vi "Autofocus.vi"() -> ()   [LabVIEW 2015]
uses:
  <vilib>/vision/Image Controls.llb/IMAQ Image.ctl
  <vilib>/Platform/TimedLoop/XDataNode/timing_clust.ctl
  <vilib>/Platform/TimedLoop/XDataNode/nitl_modes.ctl
  <vilib>/Platform/TimedLoop/XDataNode/wakeup.ctl
  <vilib>/platform/TimedLoop/XDataNode/XDataNode.xnode
  <vilib>/vision/NI_Vision_Development_Module.lvlib
  <vilib>/Platform/TimedLoop/XDataNode/XDNodeRunTimeDep.lvlib
panel:
  in  "P":dbl
  out "ImageDistances":dbl[](graph)
  out "Waveform Chart":i32(graph)
  in  "Pause?":bool
  out "decision":i32
  out "Y Resolution 2":i32
  out "X Resolution 2":i32
  out "average image buffer":T1[](array[typedef])
  out "Z autofocus distance":dbl=nan
  in  "Step size (um)":dbl
  in  "Capture BG":bool
  out "Distance":dbl=nan
  in  "Scan":bool
  out "Paused":bool
  in  "Threshold":dbl
  in  "Measure And Track":bool
  in  "Control Z":string="Off"
  out "Moving":bool
  out "error out":errorcluster
  out "Actual position":dbl[](array[numeric])=[49.9991798, 49.9997406, 53.0021973] format="%.6f"
  in  "Pi System No":i32=1
  in  "Position":cluster{"X":dbl, "Y":dbl, "Z":dbl}={"X"=50.0, "Y"=50.0, "Z"=50.0} {"Z" min=0.0 max=1000.0 step=0.001 format="%5.3g"; "Y" min=0.0 max=100.0 step=0.001 format="%06.3g"; "X" min=0.0 max=100.0 step=0.001 format="%05.3g"}
  in  "stop 2":bool
  out "Running":bool=TRUE caption="Configuration_Setup.vi is running"
  out "Conn. Axis":string[](array[string])=["1", "2", "3"]
  out "Identification":string="Physik Instrumente, E-725, 112059106, 12.01.04.04"
  in  "Z_ROI":i32[](array[numeric])=[0, 2, 10, 10]
  out "Micrograph":T1(plugin-control)
  in  "stop":bool
  # "Piezo Control"
  # "Z axis autofocus"
  # "Debug"
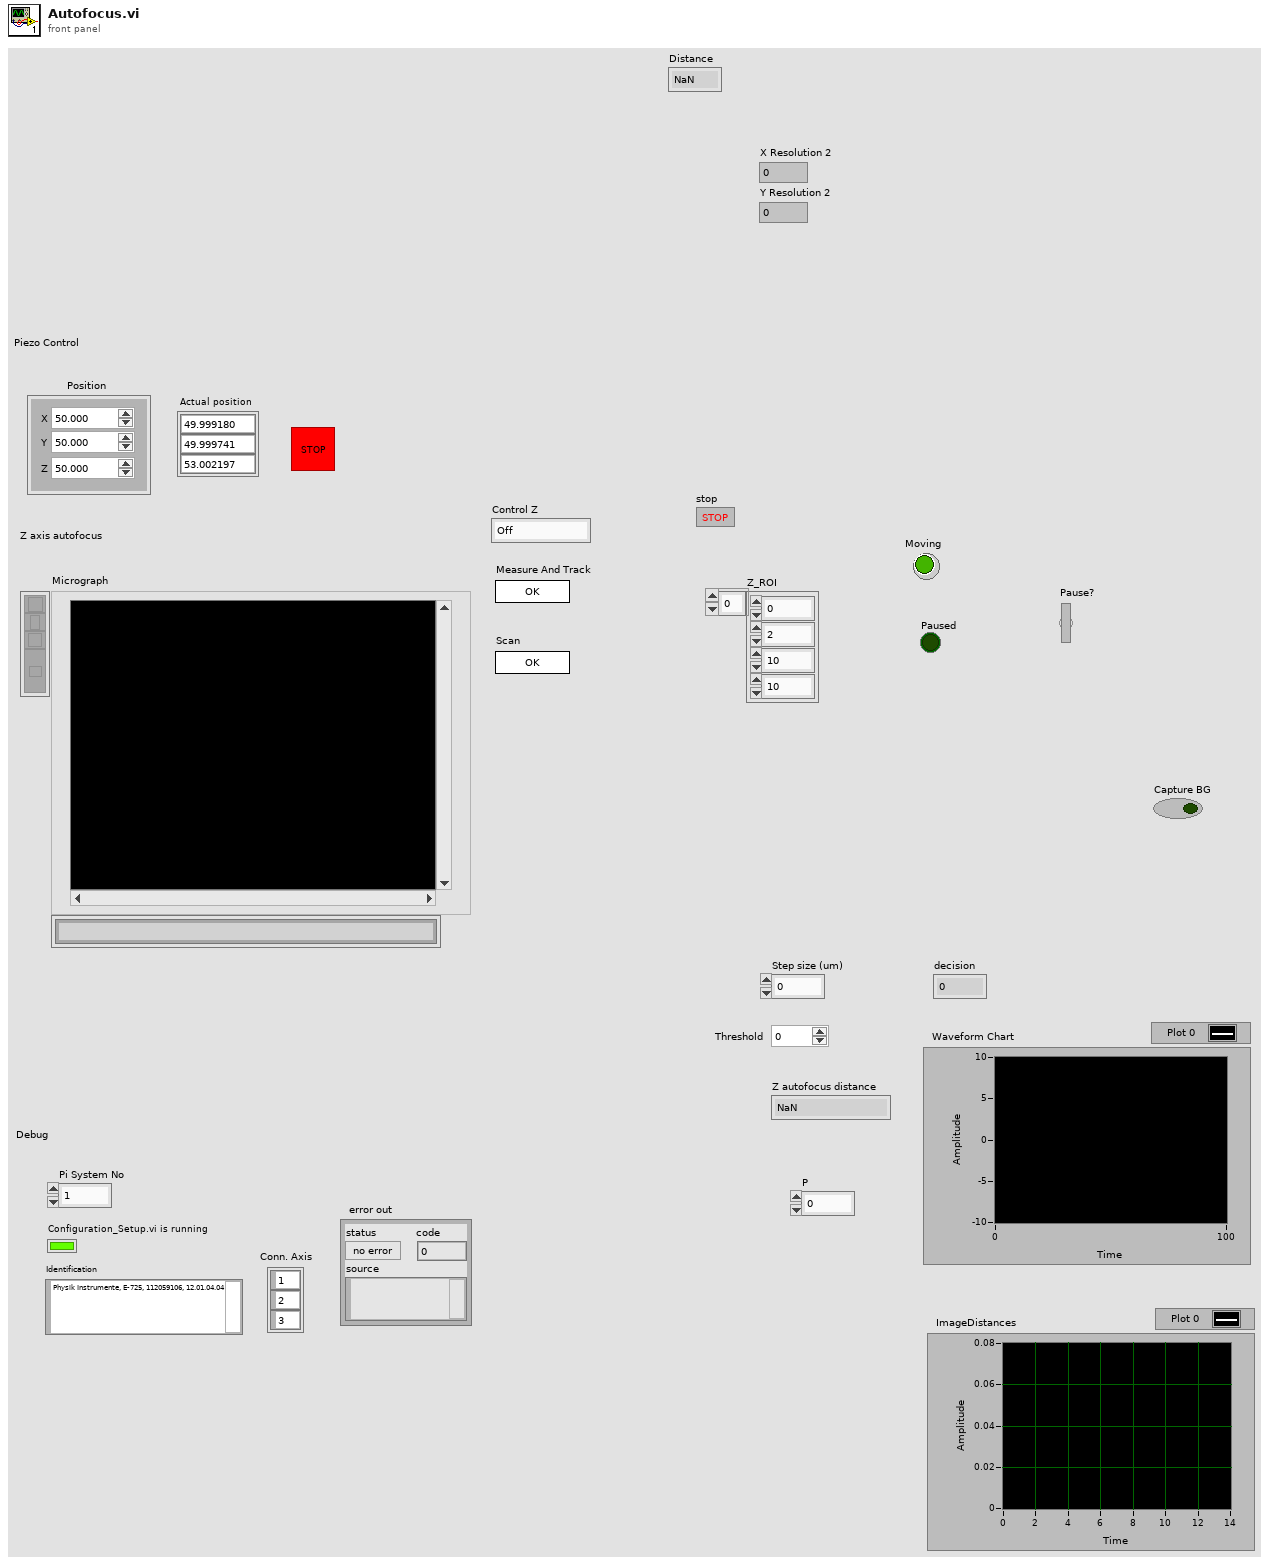
[diagram p1: front panel]
types:
  T1 = typedef "IMAQ Image.ctl" = refnum<image>
  T2 = typedef "XDNodeRunTimeDep.lvlib/timing_clust.ctl" = cluster{"Expected End [f-1]":u64, "Actual End [f-1]":u64, "Finished Late? [f-1]":bool, "Expected End [i-1]":u64, "Actual End [i-1]":u64, "Finished Late? [i-1]":bool, "Expected Start [i]":u64, "Actual Start [i]":u64, "Expected Start [f]":u64, "Actual Start [f]":u64, "Source Name":string, "Structure Name":string, "Period":i64, "Deadline":i64, "Offset":i64, "Start":i64, "Priority":i32, "Timeout":i32, "Mode":T3, "Wakeup Reason":T4, "Error":errorcluster, "Source Type":string, "Secondary Source Type":string, "Global End Time":u64, "Global Start Time":u64, "Frame Duration":u64, "Iteration Duration":u64, "Assigned CPU":i32, "I/O Scan Engine Mode":u32}
  T3 = typedef "XDNodeRunTimeDep.lvlib/nitl_modes.ctl" = enum32{"No Change", "Process missed periods, maintain original phase", "Discard missed periods, maintain original phase", "Process missed periods, ignore original phase", "Discard missed periods, ignore original phase"}
  T4 = typedef "XDNodeRunTimeDep.lvlib/wakeup.ctl" = enum32{"Normal", "Aborted", "Asynchronous wakeup", "Timing source error", "Timed loop error", "Timeout"}
  T5 = cluster{"Global Rectangle":i32[], "Contours":cluster{"Contour Type":u32, "ROI Type":u32, "Points":i32[]}[]}
  T6 = typedef "ROI Descriptor" = cluster{"Global Rectangle":i32[], "Contours":cluster{"ID":enum32{"External", "Internal"}, "Type":u32, "Coordinates":i32[]}[]}
  T7 = typedef "IMAQ Point" = cluster{"X":sgl, "Y":sgl}
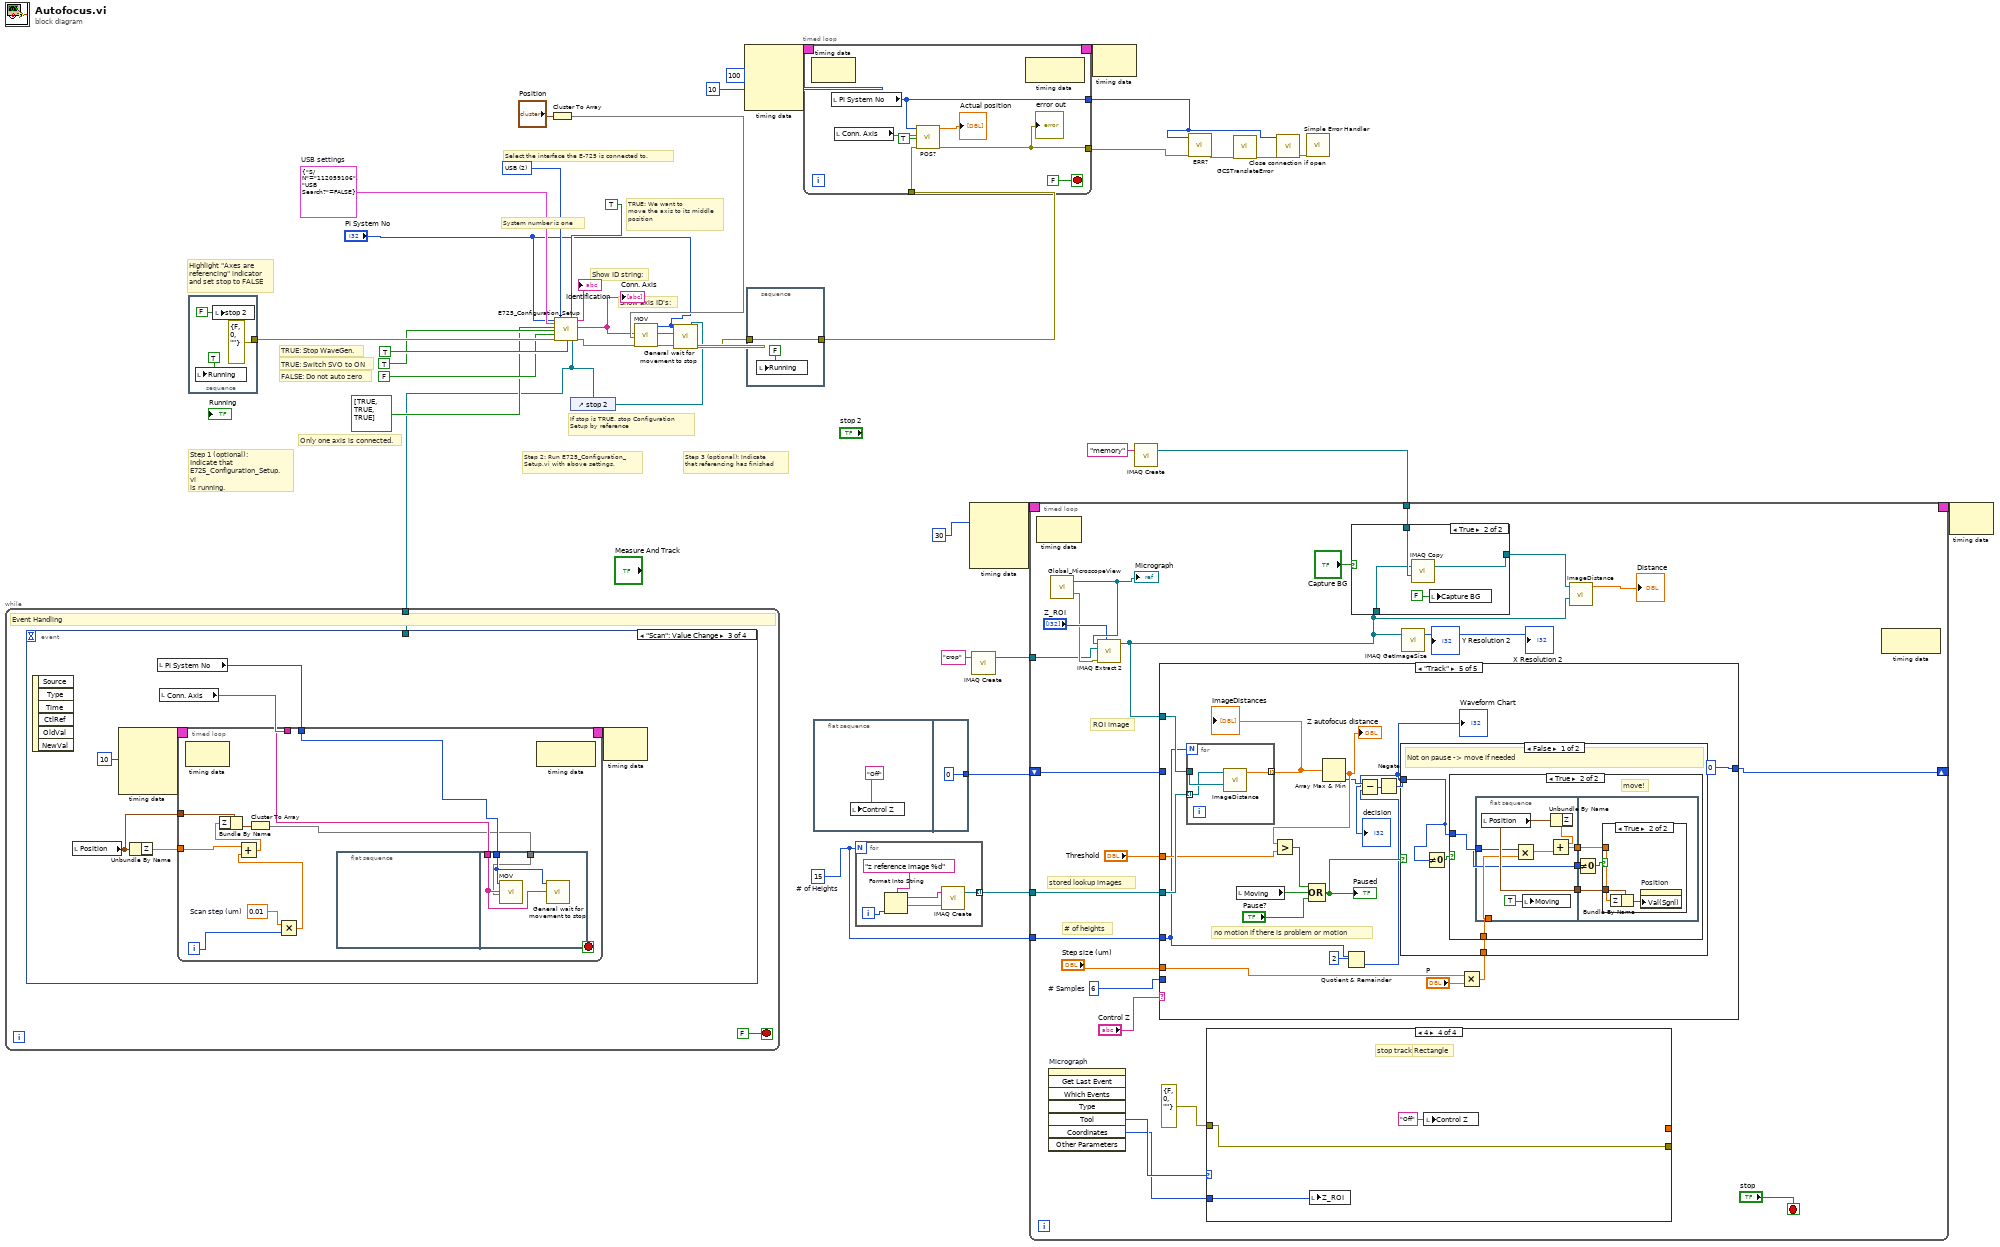
[diagram p0: block diagram]
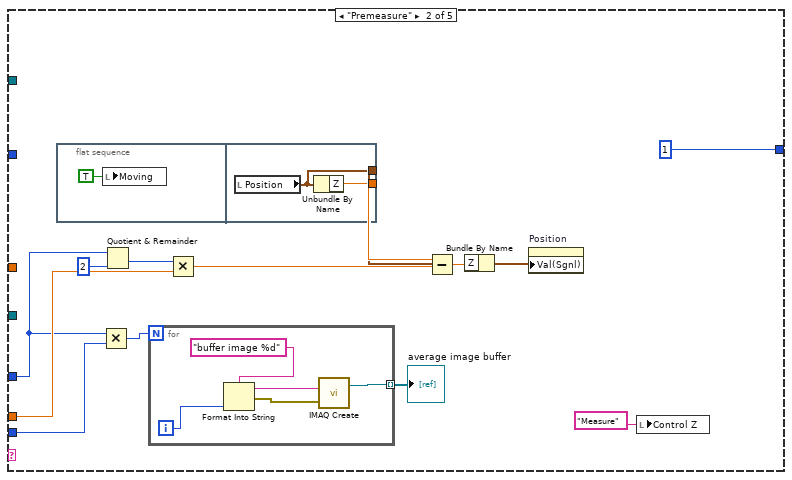
[diagram p4: hidden frame]
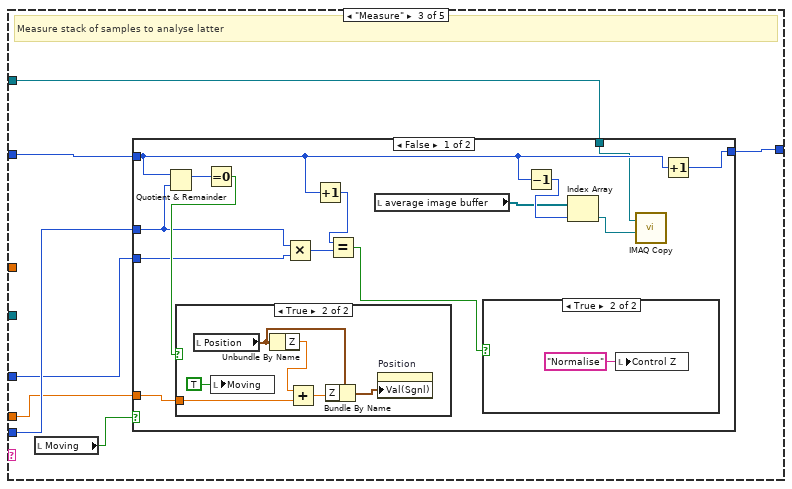
[diagram p5: hidden frame]
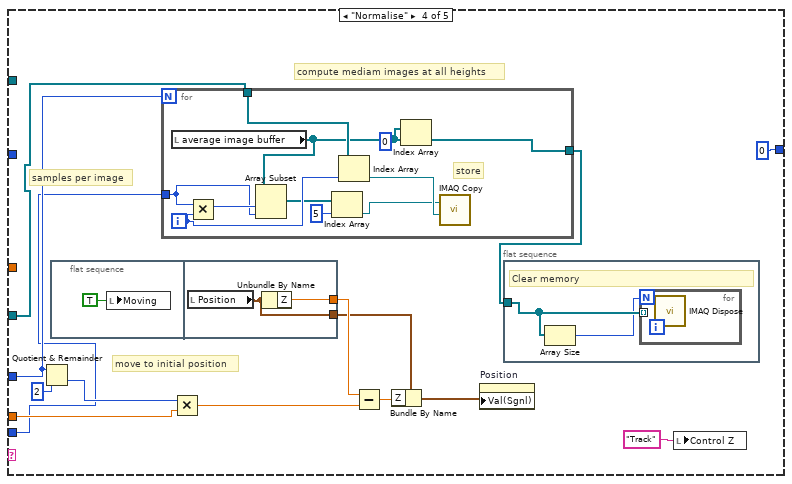
[diagram p9: hidden frame]
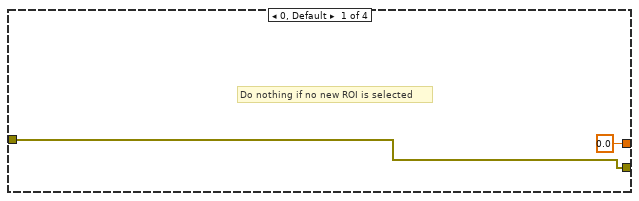
[diagram p13: hidden frame]
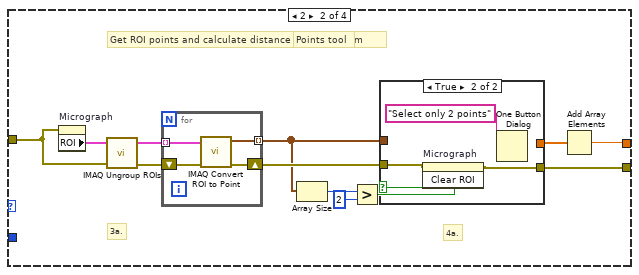
[diagram p14: hidden frame]
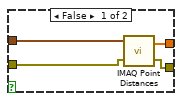
[diagram p15: hidden frame]
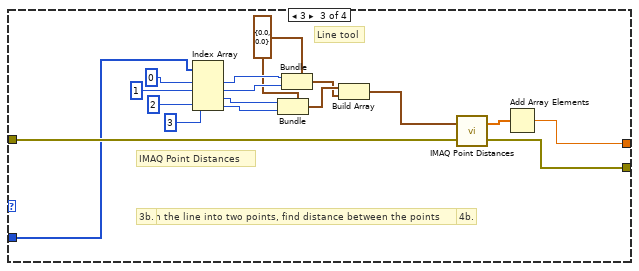
[diagram p16: hidden frame]
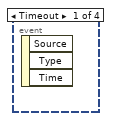
[diagram p17: hidden frame]
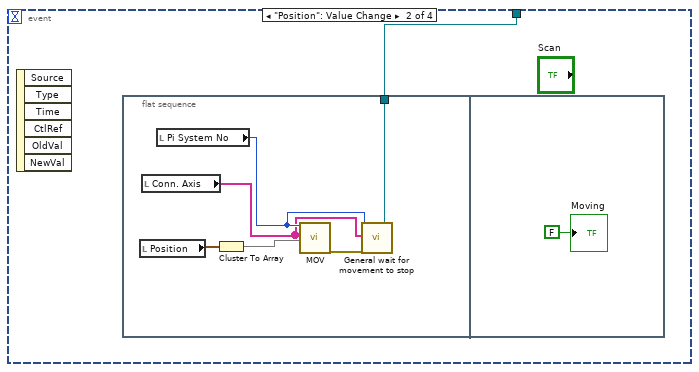
[diagram p18: hidden frame]
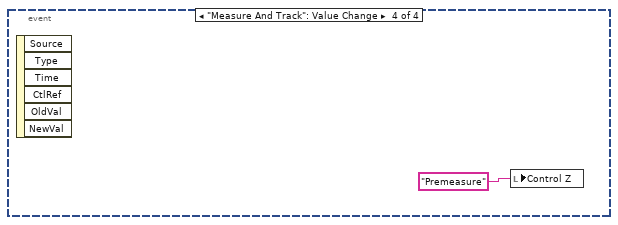
[diagram p19: hidden frame]
diagram:
  w1 = 15  # # of Heights
  w30 = cluster{"S/N":string, "USB Search?":bool} {"S/N"="112059106", "USB Search?"=FALSE}  # USB settings
  w21 = u16 2 items=["RS232", "TCP/IP", "USB"] ("Interface")
  # "Only one axis is connected."
  # "TRUE: We want to\nmove the axis to its middle\nposition"
  # "FALSE: Do not auto zero"
  # "TRUE: Switch SVO to ON"
  # "If stop is TRUE, stop Configuration\nSetup by reference"
  # "Select the interface the E-725 is connected to."
  # "Step 3 (optional): Indicate\nthat referencing has finished"
  # "Step 2: Run E725_Configuration_\nSetup.vi with above settings."
  # "Step 1 (optional): \nIndicate that\nE725_Configuration_Setup.vi\nis running."
  # "Highlight \"Axes are\nreferencing\" indicator\nand set stop to FALSE"
  # "Show axis ID's:"
  # "Show ID string:"
  # "TRUE: Stop WaveGen."
  # "System number is one"
  n1 = stacked-sequence {
    tunnel: [errorcluster {"status"=FALSE, "code"=0, "source"=""} ("error in")] -> w36
    frame #0 {
      n2 = local write "Running"(TRUE ("Running")) -> ()
      n3 = local write "stop 2"(FALSE ("stop")) -> ()
    }
  }
  n4 = Cluster To Array(cluster="Position") -> (array=w24:dbl[])
  n5 = control-ref of="stop 2"() -> (w14:refnum<vi>)
  n6 = while {
    tunnel: w14 -> [w42]
    stop <- FALSE stop-if-true
    # "Event Handling"
    n7 = event shown="[2] \"Scan\": Value Change" {
      selector: _ -> [_ _ _ _]
      dyn-events: _ -> [_ _ _ _]
      timeout: _ -> [_ _ _ _]
      tunnel: w42 -> [_ w43 _ _]
      event Timeout {
        n8 = event-data() -> ()  [unwired: 1 in, 3 out]
      }
      event "Position": Value Change {
        n9 = event-data() -> ()  [unwired: 1 in, 6 out]
        n10 = flat-sequence {
          tunnel: w43 -> [w44]
          frame #0 {
            n11 = local read "Position"() -> (w49:cluster{"X":dbl, "Y":dbl, "Z":dbl})
            n12 = local read "Conn. Axis"() -> (w45:string[])
            n13 = local read "Pi System No"() -> (w46:i32)
            n14 = Cluster To Array(cluster=w49) -> (array=w48:dbl[])
            n15 = call "MOV.vi"("System no."=w46, "Axes to move"=w45, "Position values"=w48) -> ("error out"=w47:errorcluster)  [unwired: 16 in]
            n16 = call "General wait for movement to stop.vi"("System no."=w46, "Axes to wait for"=w45, "error in"=w47, "Stop refnum"=w44) -> ()  [unwired: 14 in, 2 out]
          }
          frame #1 {
            "Moving" <- FALSE
          }
        }
      }
      event "Scan": Value Change {
        n17 = event-data() -> ()  [unwired: 1 in, 6 out]
        n18 = local read "Position"() -> (w53:cluster{"X":dbl, "Y":dbl, "Z":dbl})
        n19 = node-c288(i64 10 ("Period")) -> (w56:T2)  [unwired: 3 in]
        n20 = Unbundle By Name(w53) -> ("Z"=w57:dbl)
        n21 = local read "Pi System No"() -> (w51:i32)
        n22 = local read "Conn. Axis"() -> (w52:string[])
        n23 = timed-loop {
          tunnel: w57 -> [w65]
          timing: w56 -> [_]
          timing-out: [_] -> w55
          tunnel: w53 -> [w63]
          tunnel: w52 -> [w59]
          tunnel: w51 -> [w60]
          i -> [w66]
          stop <- _ stop-if-true
          w67 = 0.01  # Scan step (um)
          n24 = node-c288() -> ()  [unwired: 1 in, 1 out]
          n25 = Multiply(x=w67, y=w66) -> (x*y=w64:dbl)
          n26 = Add(x=w65, y=w64) -> (x+y=w61:dbl)
          n27 = Bundle By Name(cluster=w63, "Z"=w61) -> (w62:cluster{"X":dbl, "Y":dbl, "Z":dbl})
          n28 = Cluster To Array(cluster=w62) -> (array=w58:dbl[])
          n29 = flat-sequence {
            tunnel: w60 -> [w70]
            tunnel: w59 -> [w69]
            tunnel: w58 -> [w68]
            frame #0 {
            }
            frame #1 {
              n30 = call "MOV.vi"("System no."=w70, "Axes to move"=w69, "Position values"=w68) -> ()  [unwired: 16 in, 1 out]
              n31 = call "General wait for movement to stop.vi"("System no."=w70, "Axes to wait for"=w69) -> ()  [unwired: 16 in, 2 out]
            }
          }
          n32 = node-c288() -> ()  [unwired: 1 in, 1 out]
        }
        n33 = node-c288(w55) -> ()  [unwired: 1 out]
      }
      event "Measure And Track": Value Change {
        n34 = event-data() -> ()  [unwired: 1 in, 6 out]
        n35 = local write "Control Z"("Premeasure" ("Control Z")) -> ()
      }
    }
  }
  n36 = call "E725_Configuration_Setup.vi"("System no."="Pi System No", "USB settings"=w30, "Are stages connected?"=bool[] [TRUE, TRUE, TRUE], "Change servo status to ON?"=TRUE ("Use dialog to define\nconnected stages?"), "Perform autozero?"=FALSE ("Use dialog to define\nconnected stages?"), "error in"=w36, "Interface"=w21, "Stop wave generator\noutput (if any)"=TRUE ("All axes?"), "Move to middle?"=TRUE, "Stop refnum"=w14) -> ("Identification"=→"Identification":string, "All conn. axes"=w20:string[], "error out"=w26:errorcluster)  [unwired: 5 in, 2 out]
  "Conn. Axis" <- w20
  n37 = call "MOV.vi"("System no."="Pi System No", "Axes to move"=w20, "Position values"=w24, "error in"=w26) -> ("error out"=w23:errorcluster)  [unwired: 15 in]
  n38 = call "General wait for movement to stop.vi"("System no."="Pi System No", "Axes to wait for"=w20, "error in"=w23, "Stop refnum"=w14) -> ("error out"=w22:errorcluster)  [unwired: 14 in, 1 out]
  n39 = node-c288(i64 100 ("Period"), 10 ("Priority")) -> (w19:T2)  [unwired: 2 in]
  n40 = stacked-sequence {
    tunnel: w22 -> [w79]
    tunnel: [w79] -> w15
    frame #0 {
      n41 = local write "Running"(FALSE ("Running")) -> ()
    }
  }
  n42 = timed-loop {
    timing: w19 -> [_]
    timing-out: [_] -> w18
    tunnel: w15 -> [w85]
    tunnel: [w81] -> w12
    tunnel: [w80] -> w13
    stop <- FALSE stop-if-true
    n43 = node-c288() -> ()  [unwired: 1 in, 1 out]
    n44 = local read "Pi System No"() -> (w80:i32)
    n45 = local read "Conn. Axis"() -> (w84:string[])
    n46 = call "POS?.vi"("System no."=w80, "Axes to query"=w84, "All axes?"=TRUE, "error in"=w85) -> ("Position"=→"Actual position":dbl[], "error out"=w81:errorcluster)  [unwired: 14 in]
    "error out" <- w81
    n47 = node-c288() -> ()  [unwired: 1 in, 1 out]
  }
  n48 = flat-sequence {
    tunnel: [0] -> w7
    frame #0 {
      n49 = local write "Control Z"("Off" ("Control Z")) -> ()
    }
    frame #1 {
    }
  }
  n50 = for {
    N: w1 -> [_]
    tunnel: [w95] -> w3 mode=indexing
    i -> [w93]
    n51 = Format Into String(format string="z reference image %d", w93) -> (resulting string=w91:string, error out=w92:errorcluster)  [unwired: 2 in]
    n52 = call "IMAQ Create"("Image Name"=w91, "error in (no error)"=w92) -> ("New Image"=w95:T1)  [unwired: 3 in, 1 out]
  }
  n53 = node-c288(i64 30 ("Period")) -> (w10:T2)  [unwired: 3 in]
  n54 = call "IMAQ Create"("Image Name"="crop") -> ("New Image"=w2:T1)  [unwired: 4 in, 1 out]
  n55 = node-c288(w18) -> ()  [unwired: 1 out]
  n56 = call "IMAQ Create"("Image Name"="memory") -> ("New Image"=w4:T1)  [unwired: 4 in, 1 out]
  n57 = timed-loop {
    timing: w10 -> [_]
    timing-out: [_] -> w9
    shift-right: [w114] -> _
    shift-left: w7 -> [w113]
    tunnel: w4 -> [w108]
    tunnel: w3 -> [w103]
    tunnel: w2 -> [w101]
    tunnel: w1 -> [w99]
    stop <- "stop" stop-if-true
    w112 = 6  # # Samples
    # "stored lookup images"
    # "# of heights"
    # "ROI image"
    n58 = node-c288() -> ()  [unwired: 1 in, 1 out]
    n59 = invoke on="Micrograph" class="ImageControl" method="Get Last Event"() -> ("Tool"=w117:i32, "Coordinates"=w116:i32[])  [unwired: 8 in, 6 out]
    n60 = call "Global_MicroscopeView.vi"() -> ("error out"=w102:errorcluster, "MicroscopeView"=w109:T1)  [unwired: 4 in]
    "Micrograph" <- w109
    n61 = call "IMAQ Extract 2"("Optional Rectangle"="Z_ROI", "error in (no error)"=w102, "Image Dst"=w101, "Image Src"=w109) -> ("Image Dst Out"=w98:T1)  [unwired: 6 in, 1 out]
    n62 = case shown="\"Track\"" "Control Z" {
      tunnel: [w124 1 w152 0 0] -> w114
      tunnel: w113 -> [w124 _ w153 _ _]
      tunnel: w112 -> [_ w126 w151 w178 _]
      tunnel: "Step size (um)" -> [_ w135 w150 w185 w210]
      tunnel: "Threshold" -> [_ _ _ _ w221]
      tunnel: w103 -> [_ _ _ w177 w222]
      tunnel: w98 -> [_ _ w147 _ w223]
      tunnel: w99 -> [_ w125 w148 w179 w213]
      frame "Off", Default {
        # "Nothing happens"
      }
      frame "Premeasure" {
        n63 = flat-sequence {
          tunnel: [w146] -> w134
          tunnel: [w145] -> w133
          frame #0 {
            n64 = local write "Moving"(TRUE ("Moving")) -> ()
          }
          frame #1 {
            n65 = local read "Position"() -> (w145:cluster{"X":dbl, "Y":dbl, "Z":dbl})
            n66 = Unbundle By Name(w145) -> ("Z"=w146:dbl)
          }
        }
        n67 = Multiply(x=w125, y=w126) -> (x*y=w127:i32)
        n68 = Quotient & Remainder(x=w125, y=2) -> (floor(x/y)=w129:i32)  [unwired: 1 out]
        n69 = for {
          N: w127 -> [_]
          tunnel: [w143] -> w128 mode=indexing
          i -> [w141]
          n70 = Format Into String(format string="buffer image %d", w141) -> (resulting string=w140:string, error out=w142:errorcluster)  [unwired: 2 in]
          n71 = call "IMAQ Create"("Image Name"=w140, "error in (no error)"=w142) -> ("New Image"=w143:T1)  [unwired: 3 in, 1 out]
        }
        "average image buffer" <- w128
        n72 = Multiply(x=w129, y=w135) -> (x*y=w138:dbl)
        n73 = Subtract(x=w134, y=w138) -> (x-y=w137:dbl)
        n74 = Bundle By Name(cluster=w133, "Z"=w137) -> (w136:cluster{"X":dbl, "Y":dbl, "Z":dbl})
        n75 = property on="Position" class="Clust (strict)"("Val(Sgnl)"=w136) -> ()  [unwired: 2 in, 2 out]
        n76 = local write "Control Z"("Measure" ("Control Z")) -> ()
      }
      frame "Measure" {
        # "Measure stack of samples to analyse latter"
        n77 = local read "Moving"() -> (w149:bool)
        n78 = case shown="False" w149 {
          tunnel: w153 -> [w158 w175]
          tunnel: [w167 w175] -> w152
          tunnel: w151 -> [w163 _]
          tunnel: w150 -> [w164 _]
          tunnel: w148 -> [w162 _]
          tunnel: w147 -> [w155 _]
          frame False {
            n79 = Quotient & Remainder(x=w158, y=w163) -> (x-y*floor(x/y)=w166:i32)  [unwired: 1 out]
            n80 = Equal To 0?(x=w166) -> (x = 0?=w165:bool)
            n81 = case shown="True" w165 {
              tunnel: w164 -> [_ w171]
              frame False {
              }
              frame True {
                n82 = local read "Position"() -> (w174:cluster{"X":dbl, "Y":dbl, "Z":dbl})
                n83 = local write "Moving"(TRUE ("Moving")) -> ()
                n84 = Unbundle By Name(w174) -> ("Z"=w172:dbl)
                n85 = Add(x=w172, y=w171) -> (x+y=w173:dbl)
                n86 = Bundle By Name(cluster=w174, "Z"=w173) -> (w169:cluster{"X":dbl, "Y":dbl, "Z":dbl})
                n87 = property on="Position" class="Clust (strict)"("Val(Sgnl)"=w169) -> ()  [unwired: 2 in, 2 out]
              }
            }
            n88 = Multiply(x=w163, y=w162) -> (x*y=w161:i32)
            n89 = Increment(x=w158) -> (x+1=w160:i32)
            n90 = Equal?(x=w160, y=w161) -> (x = y?=w159:bool)
            n91 = local read "average image buffer"() -> (w156:T1[])
            n92 = case shown="True" w159 {
              frame False {
              }
              frame True {
                n93 = local write "Control Z"("Normalise" ("Control Z")) -> ()
              }
            }
            n94 = Decrement(x=w158) -> (x-1=w157:i32)
            n95 = Index Array(array=w156, index=w157) -> (element=w154:T1)
            n96 = call "IMAQ Copy"("Image Dst"=w154, "Image Src"=w155) -> ()  [unwired: 4 in, 2 out]
            n97 = Increment(x=w158) -> (x+1=w167:i32)
          }
          frame True {
          }
        }
      }
      frame "Normalise" {
        # "compute mediam images at all heights"
        # "samples per image"
        # "move to initial position"
        n98 = Quotient & Remainder(x=w179, y=2) -> (floor(x/y)=w180:i32)  [unwired: 1 out]
        n99 = flat-sequence {
          tunnel: [w205] -> w183
          tunnel: [w204] -> w182
          frame #0 {
            n100 = local write "Moving"(TRUE ("Moving")) -> ()
          }
          frame #1 {
            n101 = local read "Position"() -> (w204:cluster{"X":dbl, "Y":dbl, "Z":dbl})
            n102 = Unbundle By Name(w204) -> ("Z"=w205:dbl)
          }
        }
        n103 = for {
          N: w179 -> [_]
          tunnel: w178 -> [w201]
          tunnel: w177 -> [w198]
          tunnel: [w197] -> w176
          i -> [w200]
          # "store"
          n104 = local read "average image buffer"() -> (w197:T1[])
          n105 = Multiply(x=w201, y=w200) -> (x*y=w202:i32)
          n106 = Array Subset(array=w197, index=w202, length=w201) -> (w195:T1[])
          n107 = Index Array(array=w195, index=5) -> (element=w193:T1)
          n108 = Index Array(array=w198, index=w200) -> (element=w199:T1)
          n109 = Index Array(array=w197, index=0) -> ()  [unwired: 1 out]
          n110 = call "IMAQ Copy"("Image Dst"=w199, "Image Src"=w193) -> ()  [unwired: 4 in, 2 out]
        }
        n111 = Multiply(x=w180, y=w185) -> (x*y=w184:dbl)
        n112 = Subtract(x=w183, y=w184) -> (x-y=w186:dbl)
        n113 = Bundle By Name(cluster=w182, "Z"=w186) -> (w187:cluster{"X":dbl, "Y":dbl, "Z":dbl})
        n114 = property on="Position" class="Clust (strict)"("Val(Sgnl)"=w187) -> ()  [unwired: 2 in, 2 out]
        n115 = flat-sequence {
          tunnel: w176 -> [w191]
          frame #0 {
            # "Clear memory"
            n116 = Array Size(array=w191) -> (size(s)=w190:i32)
            n117 = for {
              N: w190 -> [_]
              tunnel: w191 -> [w192] mode=indexing
              n118 = call "IMAQ Dispose"("Image"=w192) -> ()  [unwired: 5 in, 1 out]
            }
          }
        }
        n119 = local write "Control Z"("Track" ("Control Z")) -> ()
      }
      frame "Track" {
        # "no motion if there is problem or motion"
        n120 = for {
          N: w213 -> [_]
          tunnel: w223 -> [w249]
          tunnel: w222 -> [w248] mode=indexing
          tunnel: [w247] -> w211 mode=indexing
          n121 = call "ImageDistance.vi"("Image 2"=w249, "Image 1"=w248) -> ("Distance"=w247:dbl)  [unwired: 9 in]
        }
        "ImageDistances" <- w211
        n122 = local read "Moving"() -> (w218:bool)
        n123 = Array Max & Min(array=w211) -> (min value=w220:dbl, min index (indices)=w215:i32)  [unwired: 2 out]
        "Z autofocus distance" <- w220
        n124 = Greater?(x=w220, y=w221) -> (0:w219:bool)
        n125 = Compound Arithmetic op=OR(w219, w218, "Pause?") -> (w216:bool)
        "Paused" <- w216
        n126 = Quotient & Remainder(x=w213, y=2) -> (floor(x/y)=w212:i32)  [unwired: 1 out]
        n127 = Subtract(x=w215, y=w212) -> (x-y=w207:i32)
        n128 = Negate(x=w207) -> (-x=w206:i32)
        "decision" <- w206
        "Waveform Chart" <- w206
        n129 = Multiply(x=w210, y="P") -> (x*y=w208:dbl)
        n130 = case shown="False" w216 {
          tunnel: w208 -> [w227 _]
          tunnel: w206 -> [w225 _]
          frame False {
            # "Not on pause -> move if needed"
            n131 = Not Equal To 0?(x=w225) -> (x != 0?=w226:bool)
            n132 = case shown="True" w226 {
              tunnel: w227 -> [_ w229]
              tunnel: w225 -> [_ w228]
              frame False {
                # "no motion needed"
              }
              frame True {
                # "move!"
                n133 = flat-sequence {
                  tunnel: [w238] -> w232
                  tunnel: [w237] -> w231
                  tunnel: w228 -> [w233]
                  tunnel: w229 -> [w235]
                  tunnel: [w233] -> w230
                  tunnel: w232 -> [w243]
                  tunnel: w231 -> [w242]
                  tunnel: w230 -> [w240]
                  frame #0 {
                    n134 = local read "Position"() -> (w238:cluster{"X":dbl, "Y":dbl, "Z":dbl})
                    n135 = Multiply(x=w233, y=w235) -> (x*y=w236:dbl)
                    n136 = local write "Moving"(TRUE ("Moving")) -> ()
                    n137 = Unbundle By Name(w238) -> ("Z"=w239:dbl)
                    n138 = Add(x=w239, y=w236) -> (x+y=w237:dbl)
                  }
                  frame #1 {
                    n139 = Not Equal To 0?(x=w240) -> (x != 0?=w241:bool)
                    n140 = case shown="True" w241 {
                      tunnel: w243 -> [_ w246]
                      tunnel: w242 -> [_ w245]
                      frame False {
                      }
                      frame True {
                        n141 = Bundle By Name(cluster=w246, "Z"=w245) -> (w244:cluster{"X":dbl, "Y":dbl, "Z":dbl})
                        n142 = property on="Position" class="Clust (strict)"("Val(Sgnl)"=w244) -> ()  [unwired: 2 in, 2 out]
                      }
                    }
                  }
                }
              }
            }
          }
          frame True {
          }
        }
      }
    }
    n143 = case shown="4" w117 {
      tunnel: w116 -> [_ _ w277 w296]
      tunnel: [w253 w258 w280 w295] -> _
      tunnel: [sgl 0.0 w256 w281 _] -> _
      tunnel: errorcluster {"status"=FALSE, "code"=0, "source"=""} ("error out") -> [w253 w255 w279 w295]
      frame 0, Default {
        # "Do nothing if no new ROI is selected"
      }
      frame 2 {
        # "Points tool"
        # "4a."
        # "3a."
        # "Get ROI points and calculate distance between them"
        n144 = property on="Micrograph" class="ImageControl"(error in=w255) -> ("ROI"=w254:T5)  [unwired: 1 in, 2 out]
        n145 = call "IMAQ Ungroup ROIs"("error in (no error)"=w255, "ROI Descriptor"=w254) -> ("error out"=w265:errorcluster, "ROI Descriptors out"=w264:T6[])  [unwired: 2 out]
        n146 = for {
          shift-right: [w273] -> w263
          shift-left: w265 -> [w276]
          tunnel: w264 -> [w275] mode=indexing
          tunnel: [w274] -> w262 mode=indexing
          n147 = call "IMAQ Convert ROI to Point"("error in (no error)"=w276, "ROI Descriptor"=w275) -> ("error out"=w273:errorcluster, "Point"=w274:T7)  [unwired: 7 out]
        }
        n148 = Array Size(array=w262) -> (size(s)=w261:i32)
        n149 = Greater?(x=w261, y=2) -> (0:w259:bool)
        n150 = case shown="True" w259 {
          tunnel: w263 -> [w269 w271]
          tunnel: w262 -> [w268 _]
          tunnel: [w267 w270] -> w258
          tunnel: [w266 _] -> w257
          frame False {
            n151 = call "IMAQ Point Distances"("Points"=w268, "error in (no error)"=w269) -> ("Distances"=w266:sgl[], "error out"=w267:errorcluster)  [unwired: 3 in]
          }
          frame True {
            n152 = invoke on="Micrograph" class="ImageControl" method="Clear ROI"(error in=w271) -> (error out=w270:errorcluster)  [unwired: 2 in, 2 out]
            n153 = One Button Dialog(message="Select only 2 points") -> ()  [unwired: 1 in, 1 out]
          }
        }
        n154 = Add Array Elements(numeric array=w257) -> (sum=w256:sgl)
      }
      frame 3 {
        w283 = cluster{"X":sgl, "Y":sgl} {"X"=0.0, "Y"=0.0}
        # "Line tool"
        # "4b."
        # "3b."
        # "Turn the line into two points, find distance between the points"
        # "IMAQ Point Distances"
        n155 = Index Array(array=w277, index #1=0 ("index"), index #2=1 ("index"), index #3=2 ("index"), index #4=3 ("index")) -> (element #1=w289:i32, element #2=w288:i32, element #3=w287:i32, element #4=w286:i32)
        n156 = Bundle(cluster=w283, "X"=w287, "Y"=w286) -> (w285:cluster{"X":sgl, "Y":sgl})
        n157 = Bundle(cluster=w283, "X"=w289, "Y"=w288) -> (w284:cluster{"X":sgl, "Y":sgl})
        n158 = Build Array(w285, w284) -> (w278:cluster{"X":sgl, "Y":sgl}[])
        n159 = call "IMAQ Point Distances"("Points"=w278, "error in (no error)"=w279) -> ("Distances"=w282:sgl[], "error out"=w280:errorcluster)  [unwired: 3 in]
        n160 = Add Array Elements(numeric array=w282) -> (sum=w281:sgl)
      }
      frame 4 {
        # "stop tracking"
        # "Rectangle"
        n161 = local write "Z_ROI"(w296) -> ()
        n162 = local write "Control Z"("Off" ("Control Z")) -> ()
      }
    }
    n163 = case shown="True" "Capture BG" {
      tunnel: w108 -> [w119 w123]
      tunnel: w98 -> [_ w122]
      tunnel: [w119 w121] -> w107
      frame False {
      }
      frame True {
        n164 = call "IMAQ Copy"("Image Dst"=w123, "Image Src"=w122) -> ("Image Dst Out"=w121:T1)  [unwired: 4 in, 1 out]
        n165 = local write "Capture BG"(FALSE ("Capture BG")) -> ()
      }
    }
    n166 = call "IMAQ GetImageSize"("Image"=w98) -> ("Y Resolution"=→"Y Resolution 2":i32, "X Resolution"=→"X Resolution 2":i32)  [unwired: 3 in, 1 out]
    n167 = call "ImageDistance.vi"("Image 2"=w98, "Image 1"=w107) -> ("Distance"=→"Distance":dbl)  [unwired: 9 in]
    n168 = node-c288() -> ()  [unwired: 1 in, 1 out]
  }
  n169 = call "ERR?.vi"("System no."=w13, "error in"=w12) -> ("error out"=w29:errorcluster)  [unwired: 16 in, 1 out]
  n170 = call "GCSTranslateError.vi"("error in"=w29) -> ("error out"=w28:errorcluster)  [unwired: 16 in, 2 out]
  n171 = call "Close connection if open.vi"("System no."=w13, "error in"=w28) -> ("error out"=w27:errorcluster)  [unwired: 16 in, 1 out]
  n172 = call <vilib>:"Simple Error Handler.vi"("error in (no error)"=w27) -> ()  [unwired: 1 in, 8 out]
  n173 = node-c288(w9) -> ()  [unwired: 1 out]
